vi "Get Alphabet Array.vi"(11 "Upper Case?":bool) -> (3 "Alphabet Array":string[](array[string]))   [LabVIEW 2020]
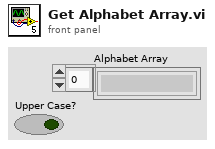
[diagram p1: front panel]
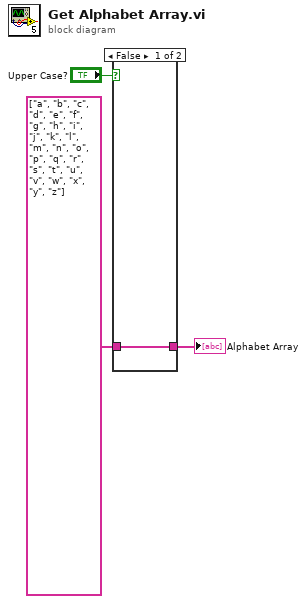
[diagram p0: block diagram]
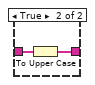
[diagram p2: hidden frame]
diagram:
  n1 = case shown="False" "Upper Case?" {
    tunnel: string[] ["a", "b", "c", "d", "e", "f", "g", "h", "i", "j", "k", "l", "m", "n", "o", "p", "q", "r", "s", "t", "u", "v", "w", "x", "y", "z"] ("name or relative path") -> [w4 w6]
    tunnel: [w4 w5] -> w1
    frame False {
    }
    frame True {
      n2 = To Upper Case(1:w6) -> (0:w5:string[])
    }
  }
  "Alphabet Array" <- w1
